vi "Engine.vi"(7 "Action":T1, 8 "error in (no error)":errorcluster, 10 "skvc in":string[](array[string]), 11 "INI Path in":path) -> (0 "error out":errorcluster, 1 "Found?":bool, 2 "skvc out":string[](array[string]), 3 "INI Path out":path)   [LabVIEW 2021, in "Config.lvlib"]
uses:
  Config.lvlib
  TypeDefs/Action.ctl
  <vilib>/Utility/error.llb/Error Cluster From Error Code.vi
  <vilib>/ErrorRing/Error Ring.xnode
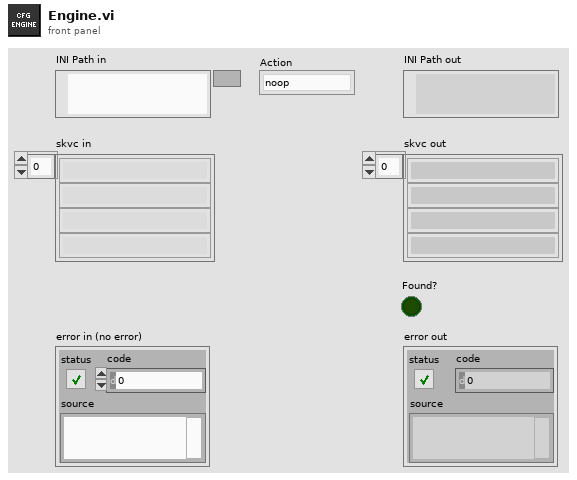
[diagram p1: front panel]
types:
  T1 = typedef "Config.lvlib/Action.ctl" = enum8{"noop", "new", "read_or_create", "read", "write", "remove", "keys", "sections", "remove_section", "import", "export", "get", "set", "pop", "add", "list", "list_sections", "pop_section"}
  T2 = cluster{"Paths":path[], "Files":cluster{"skvc":string[][]}[], "Modified":bool[], "CRC16":u16[], "PathIdx":i32, "Create":bool, "Found":bool, "skvc":string[]}
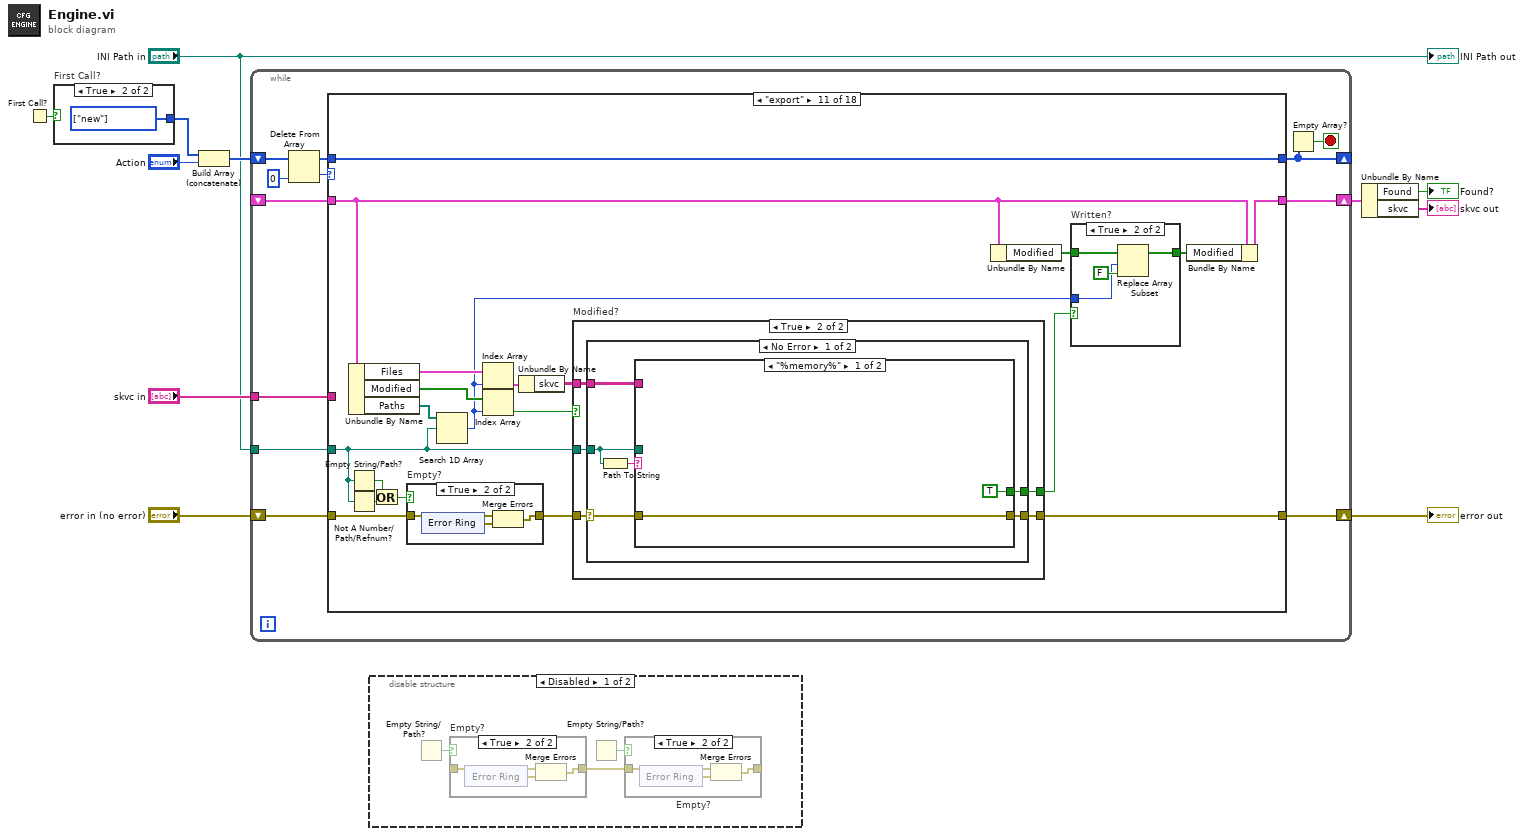
[diagram p0: block diagram]
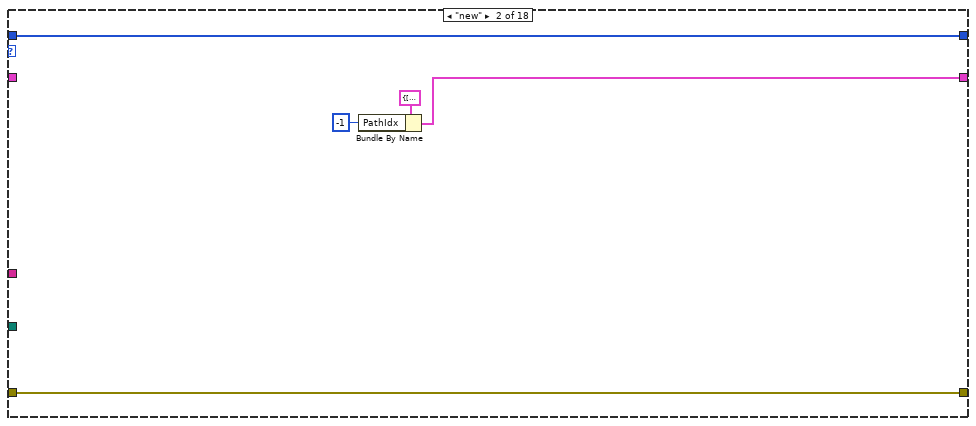
[diagram p6: hidden frame]
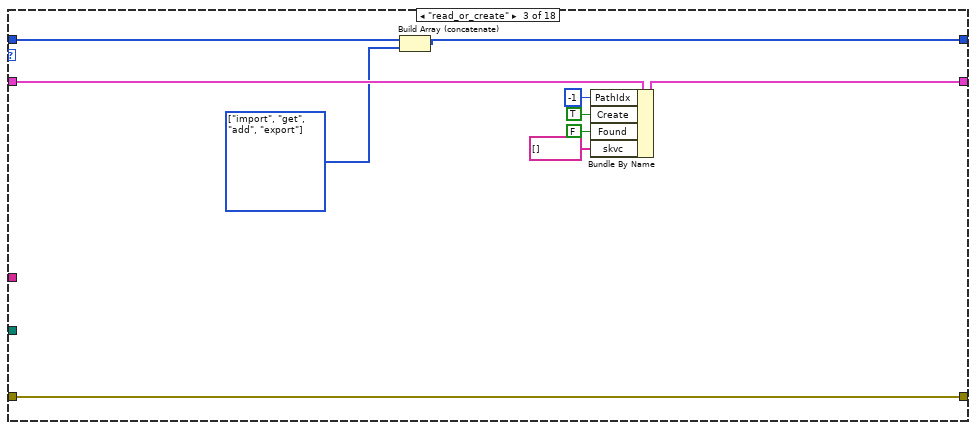
[diagram p7: hidden frame]
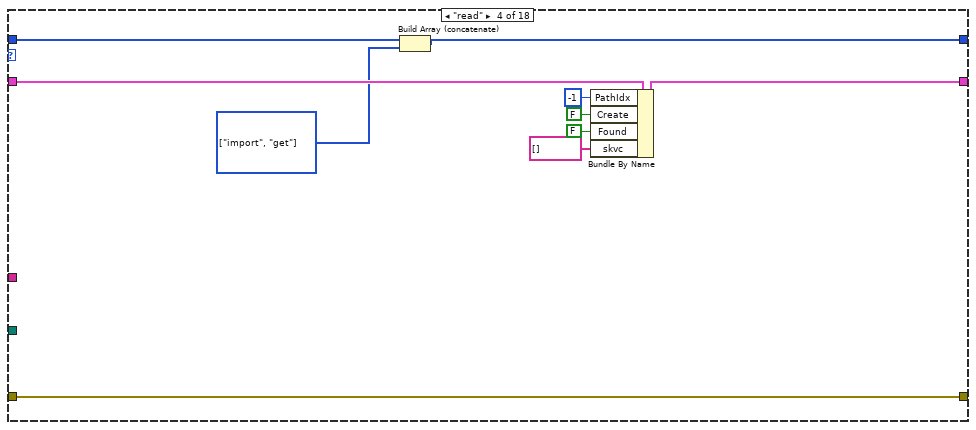
[diagram p8: hidden frame]
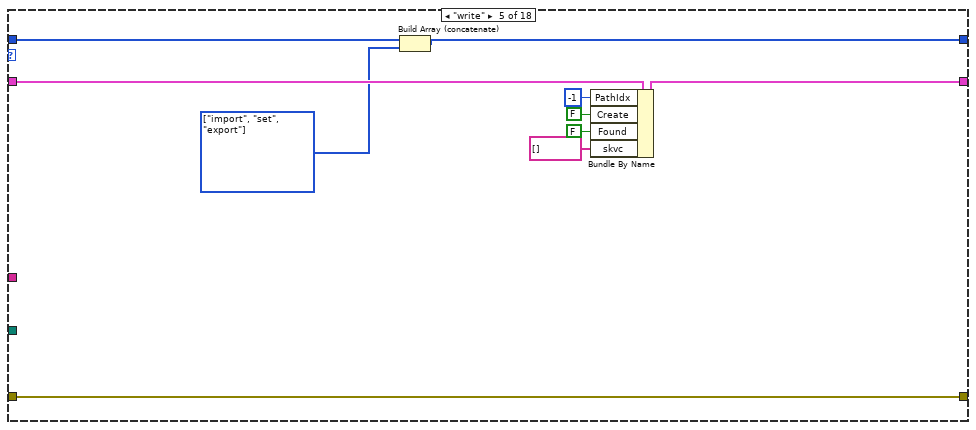
[diagram p9: hidden frame]
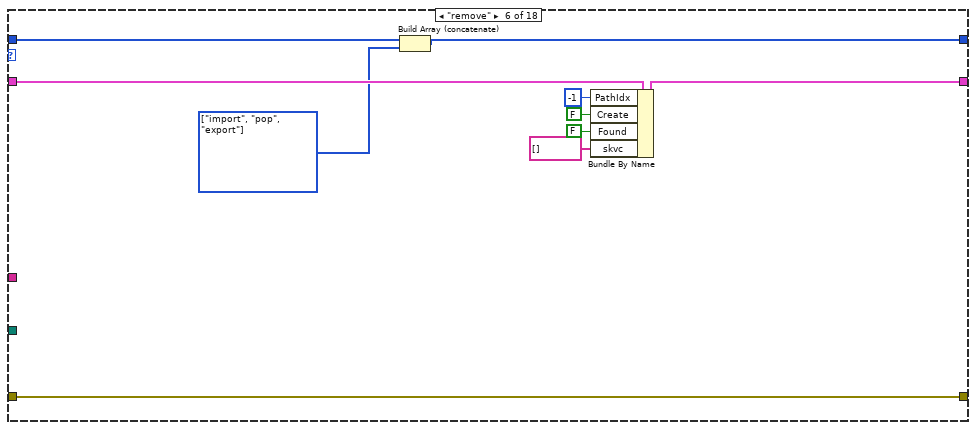
[diagram p10: hidden frame]
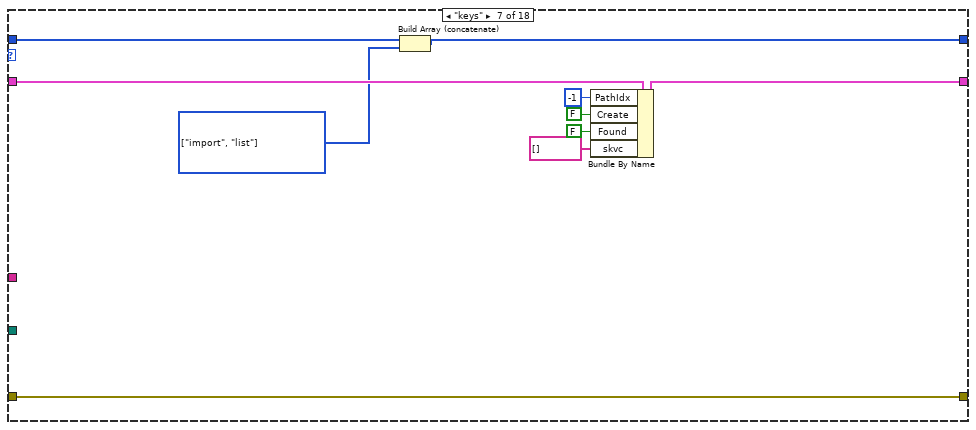
[diagram p11: hidden frame]
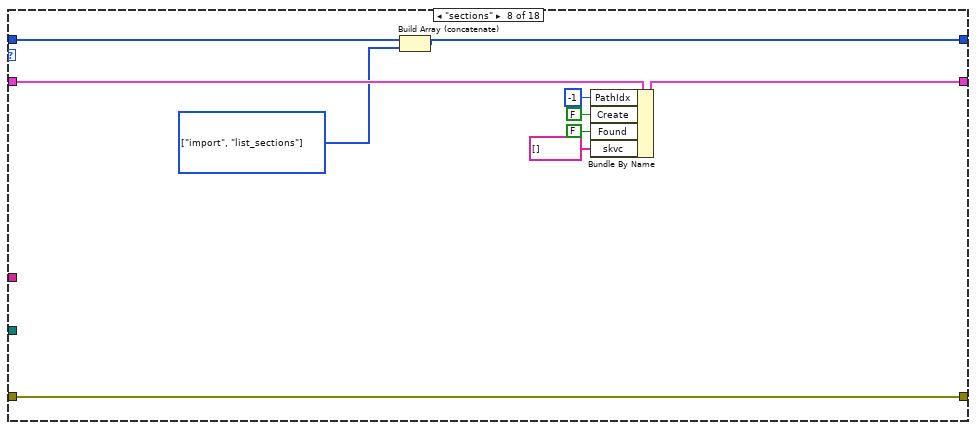
[diagram p12: hidden frame]
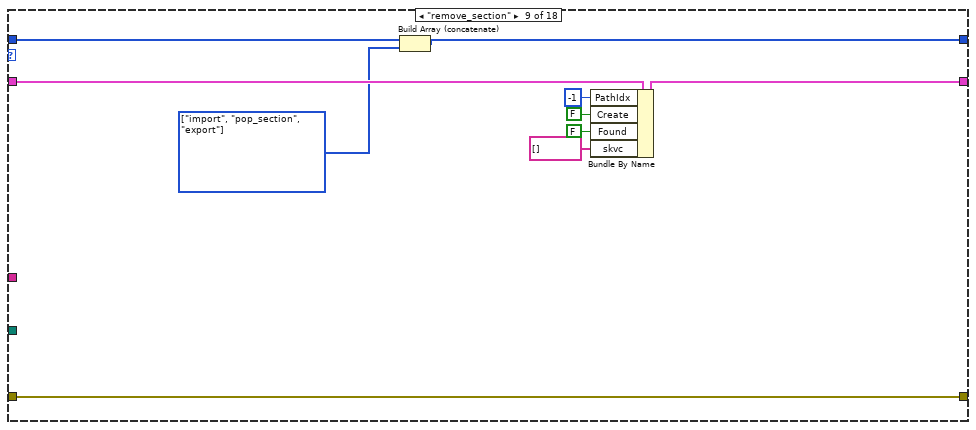
[diagram p13: hidden frame]
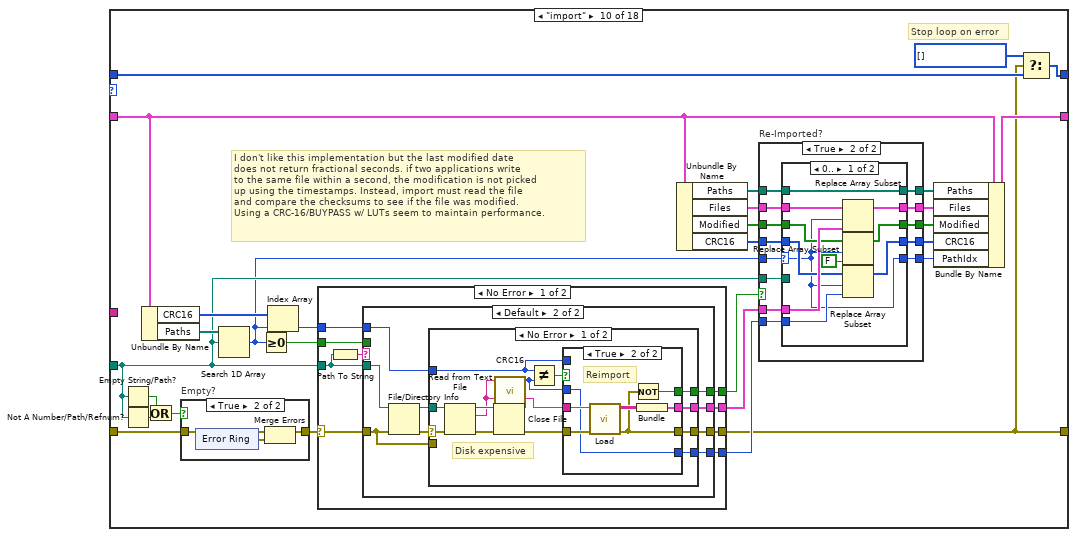
[diagram p14: hidden frame]
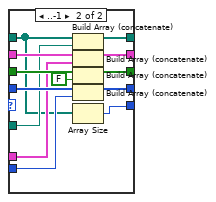
[diagram p16: hidden frame]
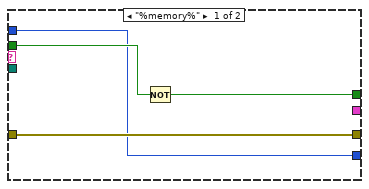
[diagram p17: hidden frame]
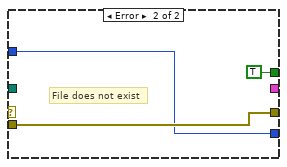
[diagram p19: hidden frame]
diagram:
  n1 = First Call?() -> (First Call?: T/F=w7:bool)
  n2 = case "First Call?" shown="True" w7 {
    tunnel: [_ w12] -> w6
    frame False {
    }
    frame True {
      w12 = T1[] [enum."new"] items=["noop", "new", "read_or_create", "read", "write", "remove", "keys", "sections", "remove_section", "import", "export", "get", "set", "pop", "add", "list", "list_sections", "pop_section"] ("appended array")
    }
  }
  n3 = Build Array (concatenate)(w6, "Action") -> (w8:T1[])
  n4 = while {
    shift-right: [w24] -> w11
    shift-left: "error in (no error)" -> [w23]
    shift-right: [w18] -> _
    shift-left: w8 -> [w22]
    shift-right: [w16] -> w3
    shift-left: _ -> [w15]
    tunnel: "INI Path in" -> [w14]
    tunnel: "skvc in" -> [w13]
    stop <- w17 stop-if-true
    n5 = Delete From Array(array=w22, index=0) -> (deleted portion=w19:T1, array with subset deleted=w21:T1[])  [unwired: 1 in]
    n6 = case shown="\"export\"" w19 {
      tunnel: [w27 w32 w34 w43 w53 w64 w74 w84 w94 w106 w240 w298 w329 w386 w430 w493 w516 w547] -> w24
      tunnel: w23 -> [w27 w32 w34 w43 w53 w64 w74 w84 w94 w130 w243 w298 w329 w386 w430 w493 w516 w547]
      tunnel: w21 -> [w26 w31 w42 w52 w62 w72 w82 w92 w102 w131 w251 w315 w332 w389 w439 w502 w523 w550]
      tunnel: [w26 w31 w33 w44 w54 w63 w73 w83 w93 w108 w251 w315 w332 w389 w439 w502 w523 w550] -> w18
      tunnel: [w25 w29 w39 w49 w59 w69 w79 w89 w99 w121 w235 w305 w330 w387 w437 w496 w517 w548] -> w16
      tunnel: w15 -> [w25 _ w41 w51 w61 w71 w81 w91 w101 w122 w237 w314 w331 w388 w438 w501 w522 w549]
      tunnel: w14 -> [_ _ _ _ _ _ _ _ _ w110 w241 _ _ _ _ _ _ _]
      tunnel: w13 -> [_ _ _ _ _ _ _ _ _ _ _ w301 w327 w379 w435 w495 _ w540]
      frame "noop" {
      }
      frame "new" {
        n7 = Bundle By Name(cluster=T2 {"Paths"=[], "Files"=[], "Modified"=[], "CRC16"=[], "PathIdx"=0, "Create"=FALSE, "Found"=FALSE, "skvc"=[]} ("StateData"), "PathIdx"=-1) -> (w29:T2)
      }
      frame "read_or_create" {
        w40 = T1[] [enum."import", enum."get", enum."add", enum."export"] items=["noop", "new", "read_or_create", "read", "write", "remove", "keys", "sections", "remove_section", "import", "export", "get", "set", "pop", "add", "list", "list_sections", "pop_section"] ("element")
        n8 = Build Array (concatenate)(w42, w40) -> (w33:T1[])
        n9 = Bundle By Name(cluster=w41, "PathIdx"=-1, "Create"=TRUE, "Found"=FALSE, "skvc"=string[] []) -> (w39:T2)
      }
      frame "read" {
        w50 = T1[] [enum."import", enum."get"] items=["noop", "new", "read_or_create", "read", "write", "remove", "keys", "sections", "remove_section", "import", "export", "get", "set", "pop", "add", "list", "list_sections", "pop_section"] ("element")
        n10 = Build Array (concatenate)(w52, w50) -> (w44:T1[])
        n11 = Bundle By Name(cluster=w51, "PathIdx"=-1, "Create"=FALSE, "Found"=FALSE, "skvc"=string[] []) -> (w49:T2)
      }
      frame "write" {
        w60 = T1[] [enum."import", enum."set", enum."export"] items=["noop", "new", "read_or_create", "read", "write", "remove", "keys", "sections", "remove_section", "import", "export", "get", "set", "pop", "add", "list", "list_sections", "pop_section"] ("element")
        n12 = Build Array (concatenate)(w62, w60) -> (w54:T1[])
        n13 = Bundle By Name(cluster=w61, "PathIdx"=-1, "Create"=FALSE, "Found"=FALSE, "skvc"=string[] []) -> (w59:T2)
      }
      frame "remove" {
        w70 = T1[] [enum."import", enum."pop", enum."export"] items=["noop", "new", "read_or_create", "read", "write", "remove", "keys", "sections", "remove_section", "import", "export", "get", "set", "pop", "add", "list", "list_sections", "pop_section"] ("element")
        n14 = Build Array (concatenate)(w72, w70) -> (w63:T1[])
        n15 = Bundle By Name(cluster=w71, "PathIdx"=-1, "Create"=FALSE, "Found"=FALSE, "skvc"=string[] []) -> (w69:T2)
      }
      frame "keys" {
        w80 = T1[] [enum."import", enum."list"] items=["noop", "new", "read_or_create", "read", "write", "remove", "keys", "sections", "remove_section", "import", "export", "get", "set", "pop", "add", "list", "list_sections", "pop_section"] ("element")
        n16 = Build Array (concatenate)(w82, w80) -> (w73:T1[])
        n17 = Bundle By Name(cluster=w81, "PathIdx"=-1, "Create"=FALSE, "Found"=FALSE, "skvc"=string[] []) -> (w79:T2)
      }
      frame "sections" {
        w90 = T1[] [enum."import", enum."list_sections"] items=["noop", "new", "read_or_create", "read", "write", "remove", "keys", "sections", "remove_section", "import", "export", "get", "set", "pop", "add", "list", "list_sections", "pop_section"] ("element")
        n18 = Build Array (concatenate)(w92, w90) -> (w83:T1[])
        n19 = Bundle By Name(cluster=w91, "PathIdx"=-1, "Create"=FALSE, "Found"=FALSE, "skvc"=string[] []) -> (w89:T2)
      }
      frame "remove_section" {
        w100 = T1[] [enum."import", enum."pop_section", enum."export"] items=["noop", "new", "read_or_create", "read", "write", "remove", "keys", "sections", "remove_section", "import", "export", "get", "set", "pop", "add", "list", "list_sections", "pop_section"] ("element")
        n20 = Build Array (concatenate)(w102, w100) -> (w93:T1[])
        n21 = Bundle By Name(cluster=w101, "PathIdx"=-1, "Create"=FALSE, "Found"=FALSE, "skvc"=string[] []) -> (w99:T2)
      }
      frame "import" {
        w107 = T1[] [] items=["noop", "new", "read_or_create", "read", "write", "remove", "keys", "sections", "remove_section", "import", "export", "get", "set", "pop", "add", "list", "list_sections", "pop_section"] ("t")
        # "I don't like this implementation but the last modified date\ndoes not return fractional seconds. if two applications write\nto the same file within a second, the modification is not picked\nup using the timestamps. Instead, import must read the file\nand compare the checksums to see if the file was modified.\nUsing a CRC-16/BUYPASS w/ LUTs seem to maintain performance."
        # "Stop loop on error"
        n22 = Empty String/Path?(string/path=w110) -> (empty?=w126:bool)
        n23 = Not A Number/Path/Refnum?(number/path/refnum=w110) -> (NaN/Path/Refnum?=w127:bool)
        n24 = Unbundle By Name(w122) -> ("CRC16"=w129:u16[], "Paths"=w123:path[])
        n25 = Or(x=w126, y=w127) -> (x .or. y?=w125:bool)
        n26 = case "Empty?" shown="True" w125 {
          tunnel: w130 -> [w223 w226]
          tunnel: [w223 w225] -> w124
          frame False {
          }
          frame True {
            n27 = xnode "Error Ring"() -> ("error out"=w224:errorcluster)
            n28 = Merge Errors(w226, w224) -> (w225:errorcluster)
          }
        }
        n29 = Search 1D Array(1D array=w123, element=w110) -> (index of element=w104:i32)  [unwired: 1 in]
        n30 = Greater Or Equal To 0?(x=w104) -> (x >= 0?=w103:bool)
        n31 = Index Array(array=w129, index=w104) -> (element=w128:u16)
        n32 = case shown="No Error" w124 {
          selector: w124 -> [w180 w222]
          tunnel: [w182 w222] -> w106
          tunnel: w128 -> [w181 w221]
          tunnel: w110 -> [w176 _]
          tunnel: [w179 _] -> w111
          tunnel: [w178 w221] -> w109
          tunnel: [w177 _] -> w112
          tunnel: w103 -> [w174 _]
          frame No Error {
            n33 = Path To String(path=w176) -> (string=w175:string)
            n34 = case shown="Default" w175 {
              tunnel: [w186 w195] -> w182
              tunnel: w181 -> [w183 w194]
              tunnel: w176 -> [_ w188]
              tunnel: w180 -> [w186 w190]
              tunnel: [_ w193] -> w179
              tunnel: [w183 w192] -> w178
              tunnel: [w184 w191] -> w177
              tunnel: w174 -> [w185 _]
              frame "%memory%" {
                n35 = Not(x=w185) -> (.not. x?=w184:bool)
              }
              frame Default {
                n36 = File/Directory Info(path=w188, error in=w190) -> (path out=w187:path, error out=w189:errorcluster)  [unwired: 5 out]
                n37 = case shown="No Error" w189 {
                  selector: w189 -> [w205 _]
                  tunnel: [w206 w220] -> w195
                  tunnel: w194 -> [w196 w218]
                  tunnel: w190 -> [_ w220]
                  tunnel: [w208 _] -> w193
                  tunnel: [w207 w218] -> w192
                  tunnel: [w204 TRUE] -> w191
                  tunnel: w187 -> [w202 _]
                  frame No Error {
                    # "Disk expensive"
                    n38 = Read from Text File(file (use dialog)=w202, error in=w205) -> (refnum out=w200:refnum<file>, text=w197:string, error out=w203:errorcluster)  [unwired: 2 in, 1 out]
                    n39 = Close File(refnum=w200, error in=w203) -> (error out=w201:errorcluster)  [unwired: 1 out]
                    n40 = call "CRC16.vi"("Data in"=w197) -> ("CRC-16"=w198:u16)  [unwired: 10 in]
                    n41 = Not Equal?(x=w196, y=w198) -> (x != y?=w199:bool)
                    n42 = case "Re-Import?" shown="True" w199 {
                      tunnel: [_ w214] -> w208
                      tunnel: [w209 w211] -> w207
                      tunnel: [w210 w216] -> w206
                      tunnel: w201 -> [w210 w213]
                      tunnel: [_ w215] -> w204
                      tunnel: w197 -> [_ w212]
                      tunnel: w198 -> [_ w211]
                      tunnel: w196 -> [w209 _]
                      frame False {
                      }
                      frame True {
                        # "Reimport"
                        n43 = call "Load.vi"("error in (no error)"=w213, "Text"=w212) -> ("error out"=w216:errorcluster, "skvc"=w217:string[][])  [unwired: 8 in]
                        n44 = Not(x=w216) -> (.not. x?=w215:bool)
                        n45 = Bundle("skvc"=w217) -> (w214:cluster{"skvc":string[][]})  [unwired: 1 in]
                      }
                    }
                  }
                  frame Error {
                    # "File does not exist"
                  }
                }
              }
            }
          }
          frame Error {
          }
        }
        n46 = Unbundle By Name(w122) -> ("Paths"=w120:path[], "Files"=w119:cluster{"skvc":string[][]}[], "Modified"=w118:bool[], "CRC16"=w117:u16[])
        n47 = case "Re-Imported?" shown="True" w112 {
          tunnel: w120 -> [w136 w149]
          tunnel: w119 -> [w135 w148]
          tunnel: w118 -> [w134 w147]
          tunnel: w117 -> [w133 w146]
          tunnel: [w133 w145] -> w116
          tunnel: [w134 w144] -> w115
          tunnel: [w135 w143] -> w114
          tunnel: [w136 w142] -> w113
          tunnel: w111 -> [_ w141]
          tunnel: w110 -> [_ w140]
          tunnel: w109 -> [_ w139]
          tunnel: w104 -> [w132 w138]
          tunnel: [w132 w137] -> w105
          frame False {
          }
          frame True {
            n48 = case shown="0.." w138 {
              selector: w138 -> [w151 _]
              tunnel: w149 -> [w160 w162]
              tunnel: w148 -> [w159 w173]
              tunnel: w147 -> [w153 w172]
              tunnel: w146 -> [w155 w171]
              tunnel: [w154 w170] -> w145
              tunnel: [w152 w169] -> w144
              tunnel: [w158 w168] -> w143
              tunnel: [w160 w167] -> w142
              tunnel: w141 -> [w157 w166]
              tunnel: w140 -> [_ w165]
              tunnel: w139 -> [w156 w163]
              tunnel: [w151 w161] -> w137
              frame 0.. {
                n49 = Replace Array Subset(array=w159, new element=w157, index=w151) -> (w158:cluster{"skvc":string[][]}[])
                n50 = Replace Array Subset(array=w153, new element=FALSE ("new element/subarray"), index=w151) -> (w152:bool[])
                n51 = Replace Array Subset(array=w155, new element=w156, index=w151) -> (w154:u16[])
              }
              frame ..-1 {
                n52 = Build Array (concatenate)(w162, w165) -> (w167:path[])
                n53 = Build Array (concatenate)(w173, w166) -> (w168:cluster{"skvc":string[][]}[])
                n54 = Build Array (concatenate)(w172, FALSE ("Boolean")) -> (w169:bool[])
                n55 = Build Array (concatenate)(w171, w163) -> (w170:u16[])
                n56 = Array Size(array=w162) -> (size(s)=w161:i32)
              }
            }
          }
        }
        n57 = Bundle By Name(cluster=w122, "Paths"=w113, "Files"=w114, "Modified"=w115, "CRC16"=w116, "PathIdx"=w105) -> (w121:T2)
        n58 = Select(t=w107, s=w106, f=w131) -> (s? t:f=w108:T1[])
      }
      frame "export" {
        n59 = Unbundle By Name(w237) -> ("Files"=w248:cluster{"skvc":string[][]}[], "Modified"=w249:bool[], "Paths"=w250:path[])
        n60 = Empty String/Path?(string/path=w241) -> (empty?=w246:bool)
        n61 = Not A Number/Path/Refnum?(number/path/refnum=w241) -> (NaN/Path/Refnum?=w247:bool)
        n62 = Or(x=w246, y=w247) -> (x .or. y?=w245:bool)
        n63 = case "Empty?" shown="True" w245 {
          tunnel: w243 -> [w288 w291]
          tunnel: [w288 w290] -> w244
          frame False {
          }
          frame True {
            n64 = xnode "Error Ring"() -> ("error out"=w289:errorcluster)
            n65 = Merge Errors(w291, w289) -> (w290:errorcluster)
          }
        }
        n66 = Search 1D Array(1D array=w250, element=w241) -> (index of element=w232:i32)  [unwired: 1 in]
        n67 = Index Array(array=w248, index=w232) -> (element=w242:cluster{"skvc":string[][]})
        n68 = Index Array(array=w249, index=w232) -> (element=w239:bool)
        n69 = Unbundle By Name(w242) -> ("skvc"=w238:string[][])
        n70 = case "Modified?" shown="True" w239 {
          tunnel: w244 -> [w257 w262]
          tunnel: w241 -> [_ w261]
          tunnel: [w257 w260] -> w240
          tunnel: w238 -> [_ w259]
          tunnel: [_ w258] -> w233
          frame False {
          }
          frame True {
            n71 = case shown="No Error" w262 {
              selector: w262 -> [w268 w287]
              tunnel: w261 -> [w264 _]
              tunnel: [w267 w287] -> w260
              tunnel: w259 -> [w265 _]
              tunnel: [w266 _] -> w258
              frame No Error {
                n72 = Path To String(path=w264) -> (string=w263:string)
                n73 = case shown="\"%memory%\"" w263 {
                  tunnel: w268 -> [w270 w283]
                  tunnel: w264 -> [_ w278]
                  tunnel: [w270 w272] -> w267
                  tunnel: [TRUE w276] -> w266
                  tunnel: w265 -> [_ w273]
                  frame "%memory%" {
                  }
                  frame Default {
                    n74 = Strip Path(path=w278) -> (stripped path=w281:path)  [unwired: 1 out]
                    n75 = File/Directory Info(path=w281, error in=w283) -> (path out=w280:path, error out=w282:errorcluster)  [unwired: 5 out]
                    n76 = case shown="Error .." w282 {
                      selector: w282 -> [w284 _]
                      tunnel: [w284 w286] -> w275
                      tunnel: w280 -> [_ w285]
                      frame No Error {
                      }
                      frame Error {
                        n77 = Create Folder(path (use dialog)=w285) -> (error out=w286:errorcluster)  [unwired: 2 in, 2 out]
                      }
                    }
                    n78 = call "Dump.vi"("error in (no error)"=w275, "skvc"=w273) -> ("error out"=w274:errorcluster, "Text"=w271:string)  [unwired: 8 in]
                    n79 = Write to Text File(file (use dialog)=w278, text=w271, error in=w274) -> (refnum out=w277:refnum<file>, error out=w279:errorcluster)  [unwired: 1 in, 1 out]
                    n80 = Close File(refnum=w277, error in=w279) -> (error out=w272:errorcluster)  [unwired: 1 out]
                    n81 = Not(x=w272) -> (.not. x?=w276:bool)
                  }
                }
              }
              frame Error {
              }
            }
          }
        }
        n82 = Unbundle By Name(w237) -> ("Modified"=w236:bool[])
        n83 = case "Written?" shown="True" w233 {
          tunnel: w236 -> [w252 w256]
          tunnel: w232 -> [_ w254]
          tunnel: [w252 w253] -> w234
          frame False {
          }
          frame True {
            n84 = Replace Array Subset(array=w256, new element=FALSE ("new element/subarray"), index=w254) -> (w253:bool[])
          }
        }
        n85 = Bundle By Name(cluster=w237, "Modified"=w234) -> (w235:T2)
      }
      frame "get" {
        # "0: Section\n1: Key"
        n86 = Unbundle By Name(w314) -> ("Files"=w313:cluster{"skvc":string[][]}[], "PathIdx"=w312:i32)
        n87 = Index Array(array=w313, index=w312) -> (element=w311:cluster{"skvc":string[][]})
        n88 = Unbundle By Name(w311) -> ("skvc"=w306:string[][])
        n89 = for {
          tunnel: w306 -> [w321] mode=indexing
          tunnel: [w318] -> w310 mode=indexing
          n90 = Index Array(array=w321) -> (element #1=w320:string, element #2=w319:string)  [unwired: 2 in]
          n91 = To Upper Case(1:w320) -> (0:w316:string)
          n92 = To Upper Case(1:w319) -> (0:w317:string)
          n93 = Bundle(w316, w317) -> (w318:cluster{string, string})  [unwired: 1 in]
        }
        n94 = Index Array(array=w301) -> (element #1=w300:string, element #2=w299:string)  [unwired: 2 in]
        n95 = To Upper Case(1:w300) -> (0:w309:string)
        n96 = To Upper Case(1:w299) -> (0:w308:string)
        n97 = Bundle(w309, w308) -> (w307:cluster{string, string})  [unwired: 1 in]
        n98 = Search 1D Array(1D array=w310, element=w307) -> (index of element=w304:i32)  [unwired: 1 in]
        n99 = Greater Or Equal To 0?(x=w304) -> (x >= 0?=w297:bool)
        n100 = Index Array(array=w306, index (row)=w304) -> (element=w303:string[])  [unwired: 1 in]
        n101 = Select(t=w303, s=w297, f=w301) -> (s? t:f=w302:string[])
        n102 = Bundle By Name(cluster=w314, "skvc"=w302, "Found"=w297) -> (w305:T2)
      }
      frame "set" {
        n103 = Unbundle By Name(w331) -> ("Modified"=w324:bool[], "Files"=w328:cluster{"skvc":string[][]}[], "PathIdx"=w325:i32)
        n104 = in-place {
          in-place-border: w327 -> [w338]
          in-place-border: [w333] -> w322
          n105 = in-place-array #1(w324, w325) -> (w335:bool)
          n106 = in-place-array #2(w328, w325) -> (w337:cluster{"skvc":string[][]})
          n107 = in-place {
            in-place-border: w338 -> [w342]
            in-place-border: w335 -> [w341]
            in-place-border: [w340] -> w334
            in-place-border: [w339] -> w333
            # "0: Section\n1: Key"
            n108 = in-place-cluster #3(w337) -> ("skvc"=w344:string[][])
            n109 = for {
              tunnel: w344 -> [w377] mode=indexing
              tunnel: [w374] -> w351 mode=indexing
              n110 = Index Array(array=w377) -> (element #1=w376:string, element #2=w375:string)  [unwired: 2 in]
              n111 = To Upper Case(1:w376) -> (0:w372:string)
              n112 = To Upper Case(1:w375) -> (0:w373:string)
              n113 = Bundle(w372, w373) -> (w374:cluster{string, string})  [unwired: 1 in]
            }
            n114 = Index Array(array=w342) -> (element #1=w347:string, element #2=w346:string)  [unwired: 2 in]
            n115 = To Upper Case(1:w347) -> (0:w350:string)
            n116 = To Upper Case(1:w346) -> (0:w349:string)
            n117 = Bundle(w350, w349) -> (w348:cluster{string, string})  [unwired: 1 in]
            n118 = Search 1D Array(1D array=w351, element=w348) -> (index of element=w345:i32)  [unwired: 1 in]
            n119 = case shown="0.." w345 {
              selector: w345 -> [w356 _]
              tunnel: w344 -> [w359 w371]
              tunnel: [w357 w370] -> w343
              tunnel: w342 -> [w355 w369]
              tunnel: w341 -> [w354 _]
              tunnel: [w353 w368] -> w340
              tunnel: [w352 w367] -> w339
              frame 0.. {
                w352 = TRUE  # Found?
                n120 = in-place {
                  in-place-border: w355 -> [w366]
                  in-place-border: w354 -> [w363]
                  in-place-border: [w361] -> w353
                  n121 = in-place-array #4(w359, w356, 2) -> (w364:string)
                  n122 = Index Array(array=w366, index=2) -> (element=w360:string)
                  n123 = Not Equal?(x=w364, y=w360) -> (x != y?=w362:bool)
                  n124 = Or(x=w363, y=w362) -> (x .or. y?=w361:bool)
                  n125 = in-place-array #4(w360) -> (w357:string[][])  [unwired: 2 out]
                }
              }
              frame ..-1 {
                w367 = FALSE  # Found?
                w368 = TRUE  # Modified?
                n126 = Build Array (concatenate)(w371, w369) -> (w370:string[][])
              }
            }
            n127 = in-place-cluster #3("skvc"=w343) -> (w336:cluster{"skvc":string[][]})
          }
          n128 = in-place-array #1(w334) -> (w323:bool[])  [unwired: 1 out]
          n129 = in-place-array #2(w336) -> (w326:cluster{"skvc":string[][]}[])  [unwired: 1 out]
        }
        n130 = Bundle By Name(cluster=w331, "Modified"=w323, "Files"=w326, "Found"=w322, "skvc"=w327) -> (w330:T2)
      }
      frame "pop" {
        n131 = Unbundle By Name(w388) -> ("Modified"=w382:bool[], "Files"=w385:cluster{"skvc":string[][]}[], "PathIdx"=w383:i32)
        n132 = in-place {
          in-place-border: w379 -> [w396]
          in-place-border: [w391] -> w380
          in-place-border: [w390] -> w378
          n133 = in-place-array #5(w382, w383) -> (w393:bool)
          n134 = in-place-array #6(w385, w383) -> (w395:cluster{"skvc":string[][]})
          n135 = in-place {
            in-place-border: w396 -> [w398]
            in-place-border: w393 -> [w402]
            in-place-border: [w401] -> w392
            in-place-border: [w400] -> w391
            in-place-border: [w397] -> w390
            # "0: Section\n1: Key"
            n136 = in-place-cluster #7(w395) -> ("skvc"=w403:string[][])
            n137 = for {
              tunnel: w403 -> [w426] mode=indexing
              tunnel: [w423] -> w410 mode=indexing
              n138 = Index Array(array=w426) -> (element #1=w425:string, element #2=w424:string)  [unwired: 2 in]
              n139 = To Upper Case(1:w425) -> (0:w421:string)
              n140 = To Upper Case(1:w424) -> (0:w422:string)
              n141 = Bundle(w421, w422) -> (w423:cluster{string, string})  [unwired: 1 in]
            }
            n142 = Index Array(array=w398) -> (element #1=w406:string, element #2=w405:string)  [unwired: 2 in]
            n143 = To Upper Case(1:w406) -> (0:w409:string)
            n144 = To Upper Case(1:w405) -> (0:w408:string)
            n145 = Bundle(w409, w408) -> (w407:cluster{string, string})  [unwired: 1 in]
            n146 = Search 1D Array(1D array=w410, element=w407) -> (index of element=w404:i32)  [unwired: 1 in]
            n147 = case shown="0.." w404 {
              selector: w404 -> [w414 _]
              tunnel: w403 -> [w415 w419]
              tunnel: w402 -> [_ w418]
              tunnel: [w412 w418] -> w401
              tunnel: [w416 w420] -> w400
              tunnel: [w413 w419] -> w399
              tunnel: w398 -> [_ w417]
              tunnel: [w411 w417] -> w397
              frame 0.. {
                w412 = TRUE  # Modified?
                w416 = TRUE  # Found?
                n148 = Delete From Array(array=w415, index (row)=w414) -> (deleted portion=w411:string[], array with subset deleted=w413:string[][])  [unwired: 2 in]
              }
              frame ..-1 {
                w420 = FALSE  # Found?
              }
            }
            n149 = in-place-cluster #7("skvc"=w399) -> (w394:cluster{"skvc":string[][]})
          }
          n150 = in-place-array #5(w392) -> (w381:bool[])  [unwired: 1 out]
          n151 = in-place-array #6(w394) -> (w384:cluster{"skvc":string[][]}[])  [unwired: 1 out]
        }
        n152 = Bundle By Name(cluster=w388, "Modified"=w381, "Files"=w384, "Found"=w380, "skvc"=w378) -> (w387:T2)
      }
      frame "add" {
        n153 = Unbundle By Name(w438) -> ("Create"=w429:bool, "Found"=w428:bool, "Modified"=w432:bool[], "Files"=w436:cluster{"skvc":string[][]}[], "PathIdx"=w433:i32)
        n154 = Compound Arithmetic op=AND(w429, invert w428) -> (w427:bool)
        n155 = case "Create Key?" shown="True" w427 {
          tunnel: w436 -> [w440 w447]
          tunnel: w435 -> [_ w446]
          tunnel: [w440 w445] -> w434
          tunnel: w433 -> [_ w444]
          tunnel: w432 -> [w441 w443]
          tunnel: [w441 w442] -> w431
          frame False {
          }
          frame True {
            n156 = in-place {
              in-place-border: w446 -> [w452]
              n157 = in-place-array #8(w443, w444) -> (w449:bool)
              n158 = in-place-array #9(w447, w444) -> (w451:cluster{"skvc":string[][]})
              n159 = in-place {
                in-place-border: w452 -> [w455]
                in-place-border: w449 -> [w454]
                in-place-border: [w453] -> w448
                # "0: Section\n1: Key"
                n160 = in-place-cluster #10(w451) -> ("skvc"=w457:string[][])
                n161 = for {
                  tunnel: w457 -> [w488] mode=indexing
                  tunnel: [w485] -> w464 mode=indexing
                  n162 = Index Array(array=w488) -> (element #1=w487:string, element #2=w486:string)  [unwired: 2 in]
                  n163 = To Upper Case(1:w487) -> (0:w483:string)
                  n164 = To Upper Case(1:w486) -> (0:w484:string)
                  n165 = Bundle(w483, w484) -> (w485:cluster{string, string})  [unwired: 1 in]
                }
                n166 = Index Array(array=w455) -> (element #1=w460:string, element #2=w459:string)  [unwired: 2 in]
                n167 = To Upper Case(1:w460) -> (0:w463:string)
                n168 = To Upper Case(1:w459) -> (0:w462:string)
                n169 = Bundle(w463, w462) -> (w461:cluster{string, string})  [unwired: 1 in]
                n170 = Search 1D Array(1D array=w464, element=w461) -> (index of element=w458:i32)  [unwired: 1 in]
                n171 = case shown="0.." w458 {
                  selector: w458 -> [w468 _]
                  tunnel: w457 -> [w471 w482]
                  tunnel: [w469 w481] -> w456
                  tunnel: w455 -> [w467 w480]
                  tunnel: w454 -> [w466 _]
                  tunnel: [w465 w479] -> w453
                  frame 0.. {
                    n172 = in-place {
                      in-place-border: w467 -> [w478]
                      in-place-border: w466 -> [w475]
                      in-place-border: [w473] -> w465
                      n173 = in-place-array #11(w471, w468, 2) -> (w476:string)
                      n174 = Index Array(array=w478, index=2) -> (element=w472:string)
                      n175 = Not Equal?(x=w476, y=w472) -> (x != y?=w474:bool)
                      n176 = Or(x=w475, y=w474) -> (x .or. y?=w473:bool)
                      n177 = in-place-array #11(w472) -> (w469:string[][])  [unwired: 2 out]
                    }
                  }
                  frame ..-1 {
                    w479 = TRUE  # Modified?
                    n178 = Build Array (concatenate)(w482, w480) -> (w481:string[][])
                  }
                }
                n179 = in-place-cluster #10("skvc"=w456) -> (w450:cluster{"skvc":string[][]})
              }
              n180 = in-place-array #8(w448) -> (w442:bool[])  [unwired: 1 out]
              n181 = in-place-array #9(w450) -> (w445:cluster{"skvc":string[][]}[])  [unwired: 1 out]
            }
          }
        }
        n182 = Bundle By Name(cluster=w438, "Modified"=w431, "Files"=w434) -> (w437:T2)
      }
      frame "list" {
        # "0: Section\n1: Key"
        n183 = Unbundle By Name(w501) -> ("Files"=w500:cluster{"skvc":string[][]}[], "PathIdx"=w499:i32)
        n184 = Index Array(array=w495) -> (element=w494:string)  [unwired: 1 in]
        n185 = Index Array(array=w500, index=w499) -> (element=w498:cluster{"skvc":string[][]})
        n186 = To Upper Case(1:w494) -> (0:w492:string)
        n187 = Unbundle By Name(w498) -> ("skvc"=w497:string[][])
        n188 = for {
          tunnel: w497 -> [w512] mode=indexing
          tunnel: [w508] -> w491 mode=indexing if=w506
          tunnel: w492 -> [w509]
          shift-right: [w504] -> w489
          shift-left: FALSE -> [w503]
          n189 = Index Array(array=w512) -> (element #1=w511:string, element #2=w508:string)  [unwired: 2 in]
          n190 = To Upper Case(1:w511) -> (0:w510:string)
          n191 = Equal?(x=w510, y=w509) -> (x = y?=w505:bool)
          n192 = Empty String/Path?(string/path=w508) -> (empty?=w507:bool)
          n193 = Or(x=w505, y=w503) -> (x .or. y?=w504:bool)
          n194 = Compound Arithmetic op=AND(invert w507, w505) -> (w506:bool)
        }
        n195 = Bundle By Name(cluster=w501, "skvc"=w491, "Found"=w489) -> (w496:T2)
      }
      frame "list_sections" {
        # "Remove duplicate sections"
        n196 = Unbundle By Name(w522) -> ("Files"=w521:cluster{"skvc":string[][]}[], "PathIdx"=w520:i32)
        n197 = Index Array(array=w521, index=w520) -> (element=w519:cluster{"skvc":string[][]})
        n198 = Unbundle By Name(w519) -> ("skvc"=w518:string[][])
        n199 = for {
          tunnel: w518 -> [w527] mode=indexing
          shift-right: [w526] -> w513
          shift-left: string[] [] -> [w525]
          n200 = Index Array(array=w527) -> (element=w524:string)  [unwired: 1 in]
          n201 = case shown="Default" w524 {
            selector: w524 -> [_ w529]
            tunnel: [w528 w531] -> w526
            tunnel: w525 -> [w528 w530]
            frame "" {
            }
            frame Default {
              n202 = To Upper Case(1:w530) -> (0:w534:string[])
              n203 = To Upper Case(1:w529) -> (0:w533:string)
              n204 = Search 1D Array(1D array=w534, element=w533) -> (index of element=w532:i32)  [unwired: 1 in]
              n205 = case shown="..-1" w532 {
                tunnel: [w535 w537] -> w531
                tunnel: w530 -> [w535 w538]
                tunnel: w529 -> [_ w536]
                frame 0.. {
                }
                frame ..-1 {
                  n206 = Build Array (concatenate)(w538, w536) -> (w537:string[])
                }
              }
            }
          }
        }
        n207 = Bundle By Name(cluster=w522, "skvc"=w513, "Found"=FALSE) -> (w517:T2)
      }
      frame "pop_section" {
        # "Remove section"
        n208 = Unbundle By Name(w549) -> ("Modified"=w543:bool[], "Files"=w546:cluster{"skvc":string[][]}[], "PathIdx"=w544:i32)
        n209 = in-place {
          in-place-border: w540 -> [w556]
          in-place-border: [w551] -> w541
          n210 = in-place-array #12(w543, w544) -> (w553:bool)
          n211 = in-place-array #13(w546, w544) -> (w555:cluster{"skvc":string[][]})
          n212 = in-place {
            in-place-border: w556 -> [w563]
            in-place-border: w553 -> [w564]
            in-place-border: [w558] -> w552
            in-place-border: [w557] -> w551
            n213 = in-place-cluster #14(w555) -> ("skvc"=w561:string[][])
            n214 = Index Array(array=w563) -> (element=w565:string)  [unwired: 1 in]
            n215 = To Upper Case(1:w565) -> (0:w562:string)
            n216 = for {
              tunnel: w561 -> [w569] mode=indexing
              tunnel: w562 -> [w570]
              tunnel: [w569] -> w560 mode=indexing if=w568
              shift-right: [w566] -> w557
              shift-left: FALSE -> [w567]
              n217 = Index Array(array=w569) -> (element=w572:string)  [unwired: 1 in]
              n218 = To Upper Case(1:w572) -> (0:w571:string)
              n219 = Not Equal?(x=w571, y=w570) -> (x != y?=w568:bool)
              n220 = Compound Arithmetic op=OR(invert w568, w567) -> (w566:bool)
            }
            n221 = Or(x=w564, y=w557) -> (x .or. y?=w558:bool)
            n222 = in-place-cluster #14("skvc"=w560) -> (w554:cluster{"skvc":string[][]})
          }
          n223 = in-place-array #12(w552) -> (w542:bool[])  [unwired: 1 out]
          n224 = in-place-array #13(w554) -> (w545:cluster{"skvc":string[][]}[])  [unwired: 1 out]
        }
        n225 = Bundle By Name(cluster=w549, "Modified"=w542, "Files"=w545, "Found"=w541, "skvc"=string[] []) -> (w548:T2)
      }
    }
    n226 = Empty Array?(array=w18) -> (empty?=w17:bool)
  }
  "error out" <- w11
  n227 = disable-structure shown="Disabled" {
    frame Disabled {
      n228 = Empty String/Path?() -> (string/path=w577:string, empty?=w576:bool)
      n229 = case "Empty?" shown="True" w576 {
        tunnel: _ -> [w587 w590]
        tunnel: [w587 w589] -> w574
        frame False {
        }
        frame True {
          n230 = xnode "Error Ring"() -> ("error out"=w588:errorcluster)
          n231 = Merge Errors(w590, w588) -> (w589:errorcluster)
        }
      }
      n232 = Empty String/Path?() -> (string/path=w573:string, empty?=w575:bool)
      n233 = case "Empty?" shown="True" w575 {
        tunnel: w574 -> [w578 w581]
        tunnel: [w578 w580] -> _
        frame False {
        }
        frame True {
          n234 = xnode "Error Ring"() -> ("error out"=w579:errorcluster)
          n235 = Merge Errors(w581, w579) -> (w580:errorcluster)
        }
      }
    }
    frame Enabled {
    }
  }
  n236 = Unbundle By Name(w3) -> ("Found"=→"Found?":bool, "skvc"=→"skvc out":string[])
  "INI Path out" <- "INI Path in"
